vi "ReadingDataFile Message Loop.vi"(7 "error in (no error)":errorcluster, 10 "Message Queues":T1) -> (0 "error out":errorcluster, 3 "appended array":string[](array[string]))   [LabVIEW 2020, in "ReadingDataFile.lvlib"]
uses:
  ReadingDataFile.lvlib
  support/Message Queue/All Message Queues.ctl
  support/Message Queue/Message Cluster.ctl
  support/Message Queue/Enqueue Message (Single).vi
  support/Message Queue/Message Queue.lvlib
  Logging/Logging.lvlib
panel:
  out "Numeric 2":i32
  out "Numeric":i32
  out "Channel 4 value 2":string
  out "Channel 3 value 2":string
  out "Channel 2 value 2":string
  out "Channel 1 value 2":string
  out "Channel 4 value 1":string
  out "Channel 3 value 1":string
  out "Channel 2 value 1":string
  out "Channel 1 value 1":string
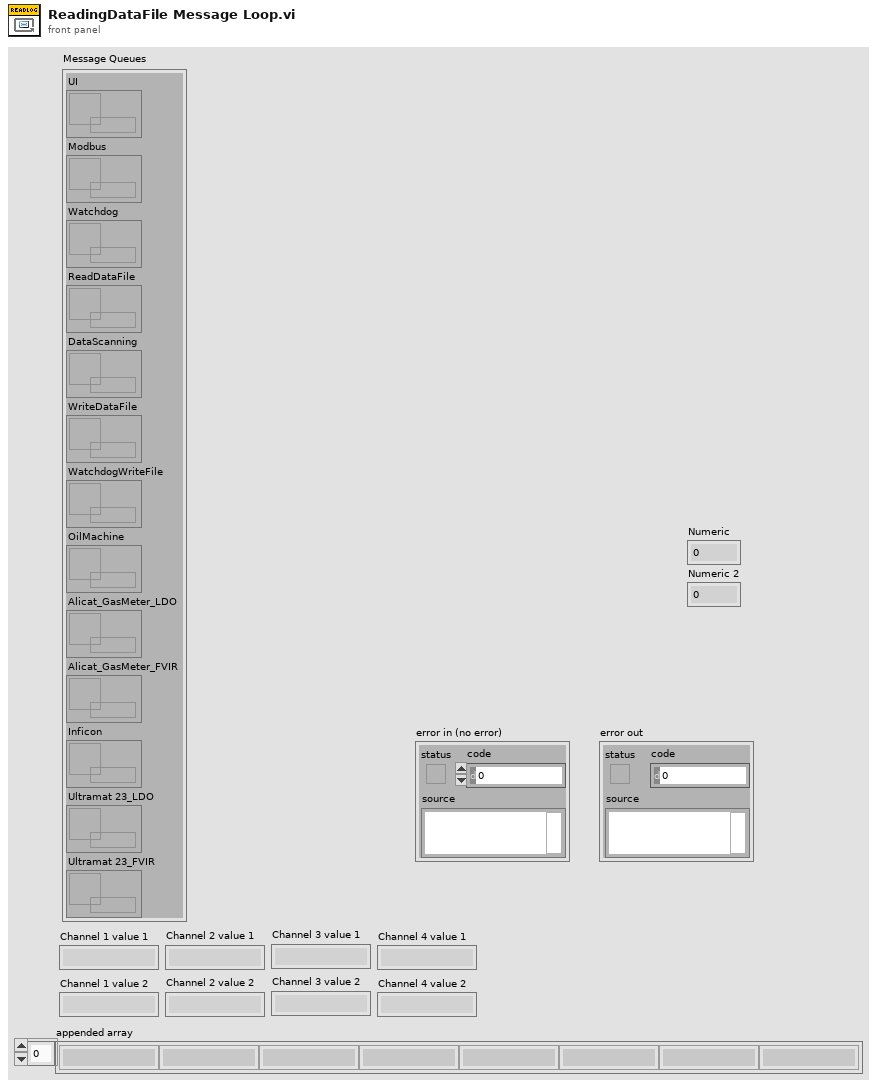
[diagram p1: front panel]
types:
  T1 = typedef "Message Queue.lvlib/All Message Queues.ctl" = cluster{"UI":refnum<queue>, "Modbus":refnum<queue>, "Watchdog":refnum<queue>, "ReadDataFile":refnum<queue>, "DataScanning":refnum<queue>, "WriteDataFile":refnum<queue>, "WatchdogWriteFile":refnum<queue>, "OilMachine":refnum<queue>, "Alicat_GasMeter_LDO":refnum<queue>, "Inficon":refnum<queue>, "Ultramat 23_LDO":refnum<queue>, "Alicat_GasMeter_FVIR":refnum<queue>, "Ultramat 23_FVIR":refnum<queue>}
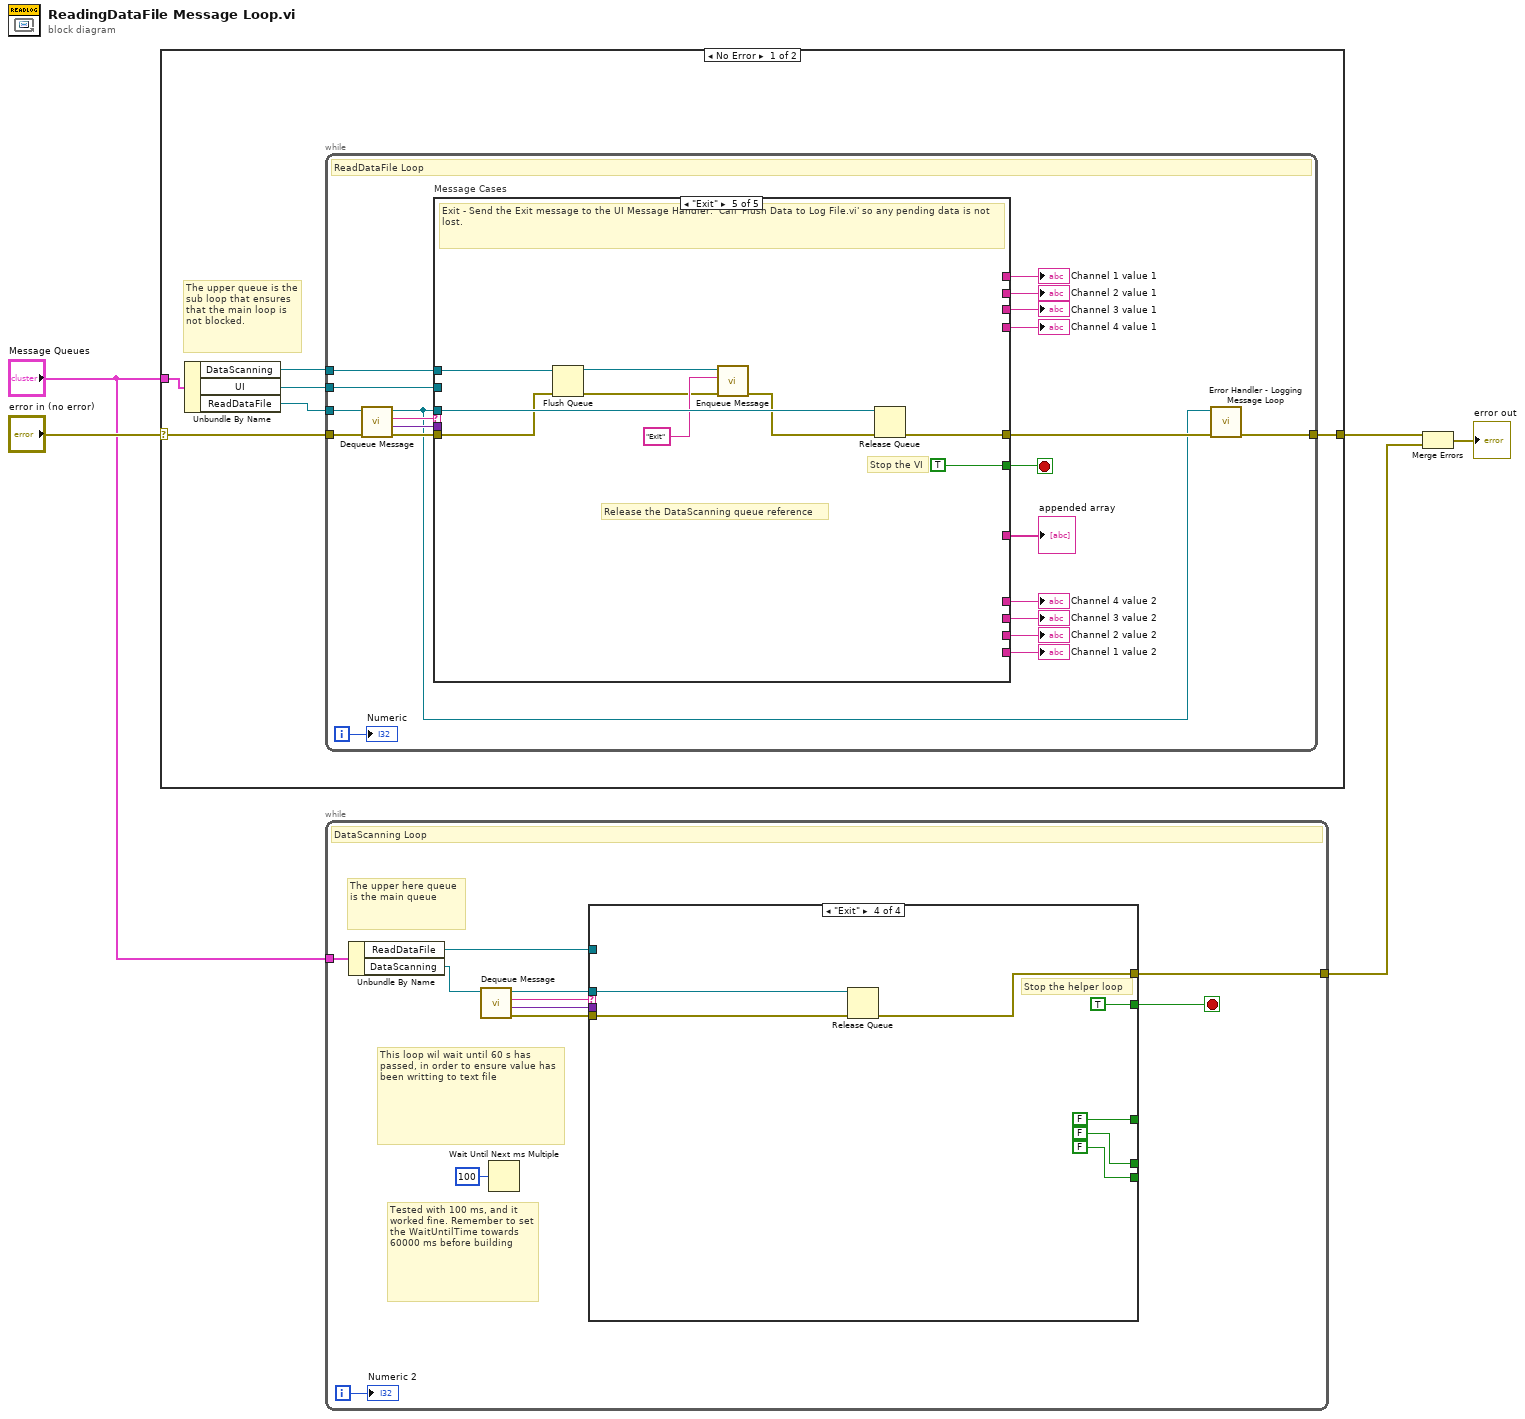
[diagram p0: block diagram]
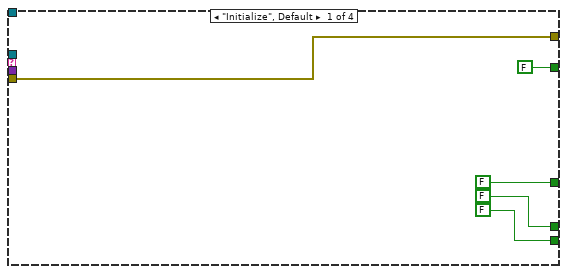
[diagram p2: hidden frame]
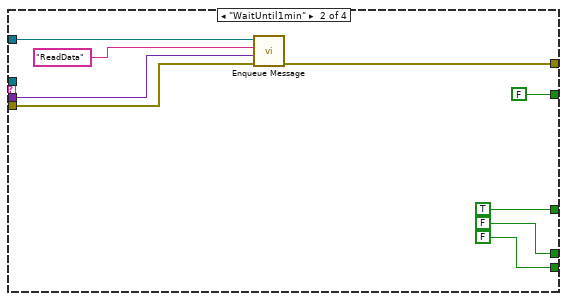
[diagram p3: hidden frame]
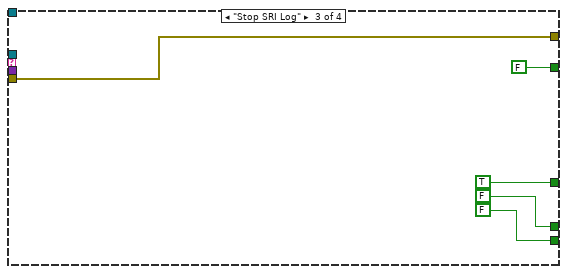
[diagram p4: hidden frame]
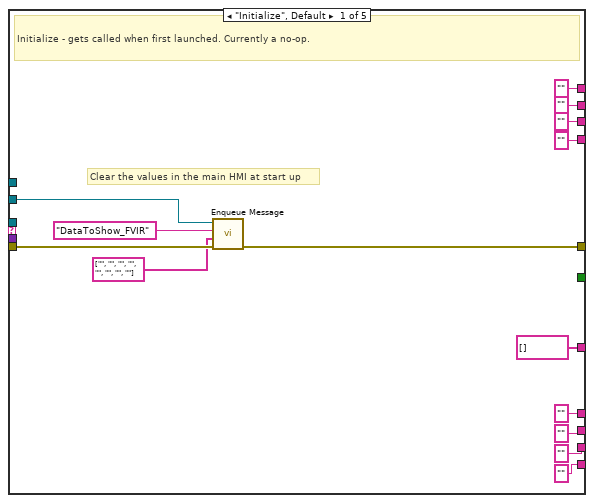
[diagram p5: hidden frame]
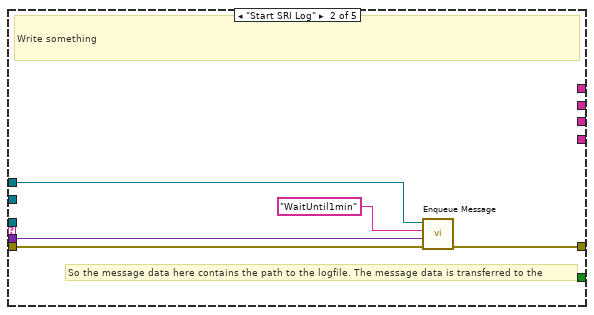
[diagram p6: hidden frame]
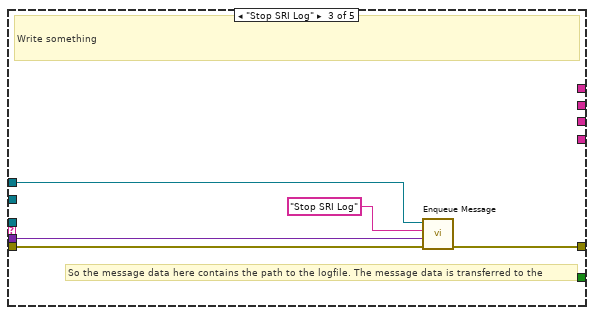
[diagram p7: hidden frame]
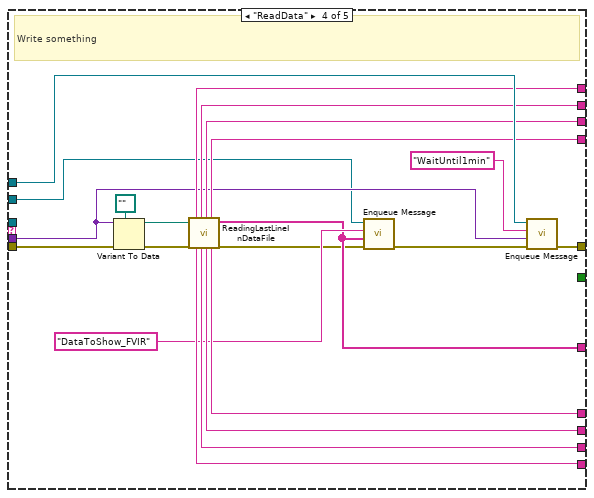
[diagram p8: hidden frame]
diagram:
  n1 = case shown="No Error" "error in (no error)" {
    selector: "error in (no error)" -> [w9 w87]
    tunnel: "Message Queues" -> [w11 _]
    tunnel: [w10 w87] -> w3
    frame No Error {
      # "The upper queue is the sub loop that ensures that the main loop is not blocked."
      n2 = Unbundle By Name(w11) -> ("DataScanning"=w8:refnum<queue>, "UI"=w6:refnum<queue>, "ReadDataFile"=w7:refnum<queue>)
      n3 = while {
        tunnel: w7 -> [w27]
        tunnel: w8 -> [w24]
        tunnel: w9 -> [w31]
        tunnel: [w26] -> w10
        tunnel: w6 -> [w13]
        i -> [w12]
        stop <- w32 stop-if-true
        # "ReadDataFile Loop"
        n4 = call "Dequeue Message.vi"("error in (no error)"=w31, "Message Queue"=w27) -> ("error out"=w30:errorcluster, "Message Data"=w28:variant, "Message"=w29:string, "dup Message Queue"=w23:refnum<queue>)  [unwired: 6 in]
        n5 = case "Message Cases" shown="\"Exit\"" w29 {
          tunnel: w23 -> [_ _ _ _ w85]
          tunnel: w30 -> [w36 w48 w53 w60 w80]
          tunnel: [w35 w51 w56 w77 w84] -> w25
          tunnel: [_ _ _ _ TRUE] -> w32
          tunnel: w28 -> [_ w47 w52 w58 _]
          tunnel: w24 -> [_ w49 w54 w75 w81]
          tunnel: [string[] [] _ _ w65 _] -> w14
          tunnel: ["" ("Channel 4 value 2") _ _ w74 _] -> w22
          tunnel: ["" ("Channel 3 value 1") _ _ w73 _] -> w21
          tunnel: ["" ("Channel 2 value 1") _ _ w72 _] -> w20
          tunnel: ["" ("Channel 1 value 1") _ _ w71 _] -> w19
          tunnel: ["" ("Channel 4 value 1") _ _ w67 _] -> w18
          tunnel: ["" ("Channel 3 value 2") _ _ w70 _] -> w17
          tunnel: ["" ("Channel 2 value 2") _ _ w69 _] -> w16
          tunnel: ["" ("Channel 1 value 2") _ _ w68 _] -> w15
          tunnel: w13 -> [w37 _ _ w57 _]
          frame "Initialize", Default {
            # "Clear the values in the main HMI at start up"
            # "Initialize - gets called when first launched. Currently a no-op."
            n6 = call-poly "Enqueue Message.vi"("error in (no error)"=w36, "Message Data"=string[] ["", "", "", "", "", "", "", ""], "Message"="DataToShow_FVIR", "Message Queue"=w37) -> ("error out"=w35:errorcluster)  [unwired: 6 in, 1 out]
          }
          frame "Start SRI Log" {
            # "So the message data here contains the path to the logfile. The message data is transferred to the"
            # "Write something"
            n7 = call-poly "Enqueue Message.vi"("error in (no error)"=w48, "Message Data"=w47, "Message"="WaitUntil1min", "Message Queue"=w49) -> ("error out"=w51:errorcluster)  [unwired: 6 in, 1 out]
          }
          frame "Stop SRI Log" {
            # "So the message data here contains the path to the logfile. The message data is transferred to the"
            # "Write something"
            n8 = call-poly "Enqueue Message.vi"("error in (no error)"=w53, "Message Data"=w52, "Message"="Stop SRI Log", "Message Queue"=w54) -> ("error out"=w56:errorcluster)  [unwired: 6 in, 1 out]
          }
          frame "ReadData" {
            # "Write something"
            n9 = Variant To Data(error in=w60, type=path "", Variant=w58) -> (data=w61:path, error out=w59:errorcluster)
            n10 = call "ReadingLastLineInDataFile.vi"("file path (dialog if empty)"=w61, "error in (no error)"=w59) -> ("Channel 1 value 1"=w71:string, "Channel 1 value 2"=w68:string, "Channel 2 value 1"=w72:string, "Channel 2 value 2"=w69:string, "Channel 3 value 1"=w73:string, "Channel 3 value 2"=w70:string, "Channel 4 value 2"=w74:string, "Channel 4 value 1"=w67:string, "Array with data values"=w65:string[], "error out"=w64:errorcluster)  [unwired: 8 in]
            n11 = call-poly "Enqueue Message.vi"("error in (no error)"=w64, "Message Data"=w65, "Message"="DataToShow_FVIR", "Message Queue"=w57) -> ("error out"=w63:errorcluster)  [unwired: 6 in, 1 out]
            n12 = call-poly "Enqueue Message.vi"("error in (no error)"=w63, "Message Data"=w58, "Message"="WaitUntil1min", "Message Queue"=w75) -> ("error out"=w77:errorcluster)  [unwired: 6 in, 1 out]
          }
          frame "Exit" {
            # "Release the DataScanning queue reference"
            # "Stop the VI"
            # "Exit - Send the Exit message to the UI Message Handler.  Call 'Flush Data to Log File.vi' so any pending data is not lost."
            n13 = Flush Queue(queue=w81, error in (no error)=w80) -> (queue out=w79:refnum<queue>, error out=w78:errorcluster)  [unwired: 1 out]
            n14 = call-poly "Enqueue Message.vi"("error in (no error)"=w78, "Message"="Exit", "Message Queue"=w79) -> ("error out"=w82:errorcluster)  [unwired: 7 in, 1 out]
            n15 = Release Queue(queue=w85, error in (no error)=w82) -> (error out=w84:errorcluster)  [unwired: 1 in, 2 out]
          }
        }
        "Channel 1 value 1" <- w19
        "Channel 2 value 1" <- w20
        "Channel 3 value 1" <- w21
        "Channel 4 value 1" <- w22
        "Channel 1 value 2" <- w15
        "Channel 2 value 2" <- w16
        "Channel 3 value 2" <- w17
        "Channel 4 value 2" <- w18
        "appended array" <- w14
        n16 = call "Error Handler - Logging Message Loop.vi"("error in (no error)"=w25, "Message Queue"=w23) -> ("dup error in"=w26:errorcluster)  [unwired: 8 in, 1 out]
        "Numeric" <- w12
      }
    }
    frame Error {
    }
  }
  n17 = while {
    tunnel: "Message Queues" -> [w98]
    tunnel: [w94] -> w2
    i -> [w88]
    stop <- w95 stop-if-true
    # "Tested with 100 ms, and it worked fine. Remember to set the WaitUntilTime towards 60000 ms before building"
    # "The upper here queue is the main queue"
    # "This loop wil wait until 60 s has passed, in order to ensure value has been writting to text file"
    # "DataScanning Loop"
    n18 = Unbundle By Name(w98) -> ("ReadDataFile"=w91:refnum<queue>, "DataScanning"=w92:refnum<queue>)
    n19 = call "Dequeue Message.vi"("Message Queue"=w92) -> ("error out"=w96:errorcluster, "Message Data"=w89:variant, "Message"=w97:string, "dup Message Queue"=w90:refnum<queue>)  [unwired: 7 in]
    n20 = Wait Until Next ms Multiple(millisecond multiple=u32 100) -> ()  [unwired: 1 out]
    n21 = case shown="\"Exit\"" w97 {
      tunnel: w96 -> [w103 w106 w113 w124]
      tunnel: [w103 w105 w113 w123] -> w94
      tunnel: [FALSE TRUE TRUE FALSE] -> _
      tunnel: [FALSE FALSE FALSE FALSE] -> _
      tunnel: [FALSE FALSE FALSE FALSE] -> _
      tunnel: [FALSE FALSE FALSE TRUE] -> w95
      tunnel: w91 -> [_ w107 _ _]
      tunnel: w90 -> [_ _ _ w118]
      tunnel: w89 -> [_ w104 _ _]
      frame "Initialize", Default {
      }
      frame "WaitUntil1min" {
        n22 = call-poly "Enqueue Message.vi"("error in (no error)"=w106, "Message Data"=w104, "Message"="ReadData", "Message Queue"=w107) -> ("error out"=w105:errorcluster)  [unwired: 6 in, 1 out]
      }
      frame "Stop SRI Log" {
      }
      frame "Exit" {
        # "Stop the helper loop"
        n23 = Release Queue(queue=w118, error in (no error)=w124) -> (error out=w123:errorcluster)  [unwired: 1 in, 2 out]
      }
    }
    "Numeric 2" <- w88
  }
  n24 = Merge Errors(w3, w2) -> (→"error out":errorcluster)
